vi "S2DS_Initial Scan parameters (SubVI).vi"(10 "Scan parameters (in)":T2 {"Y data taking" items=["in both direction", "in up direction only", "in down direction only"]; "X data taking" items=["in both direction", "in up direction only", "in down direction only"]}, 11 "WC info list":T3) -> (2 "WC Info list out":T1[](array[typedef]), 3 "Scan parameters out":T2 {"Y data taking" items=["in both direction", "in up direction only", "in down direction only"]; "X data taking" items=["in both direction", "in up direction only", "in down direction only"]})   [LabVIEW 2025]
uses:
  TYPE DEFS/S2DS_WC info.ctl
  TYPE DEFS/S2DS_Single WC info.ctl
  TYPE DEFS/S2DS_Sweep Info.ctl
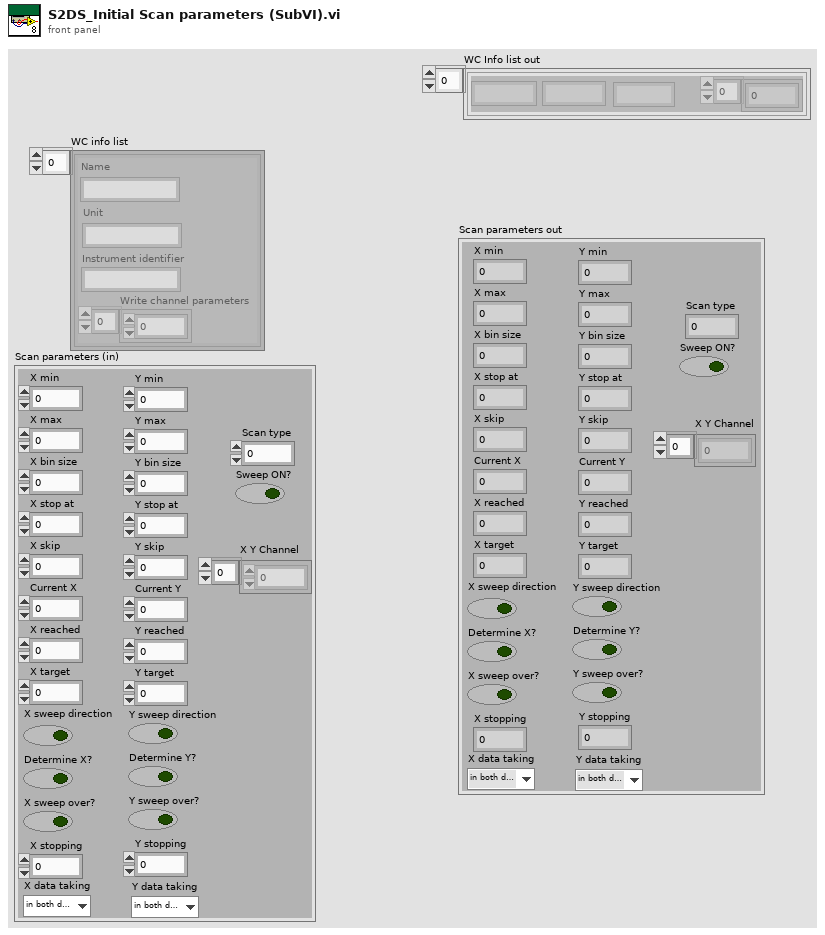
[diagram p1: front panel]
types:
  T1 = typedef "S2DS_Single WC info.ctl" = cluster{"Instrument identifier":string, "Write channel parameters":dbl[], "Name":string, "Unit":string}
  T2 = typedef "S2DS_Sweep Info.ctl" = cluster{"X min":ext, "X max":dbl, "Y min":dbl, "Y max":dbl, "X bin size":dbl, "Y bin size":dbl, "X stop at":dbl, "Y stop at":dbl, "X skip":u64, "Y skip":u64, "Current X":dbl, "Current Y":dbl, "X reached":i32, "Y reached":i32, "X target":dbl, "Y target":dbl, "Sweep ON?":bool, "X sweep direction":bool, "Y sweep direction":bool, "Determine X?":bool, "Determine Y?":bool, "X sweep over?":bool, "Y sweep over?":bool, "Scan type":i32, "X stopping":i32, "Y stopping":i32, "X Y Channel":u16[], "X data taking":u16, "Y data taking":u16}
  T3 = typedef "S2DS_WC info.ctl" = T1[]
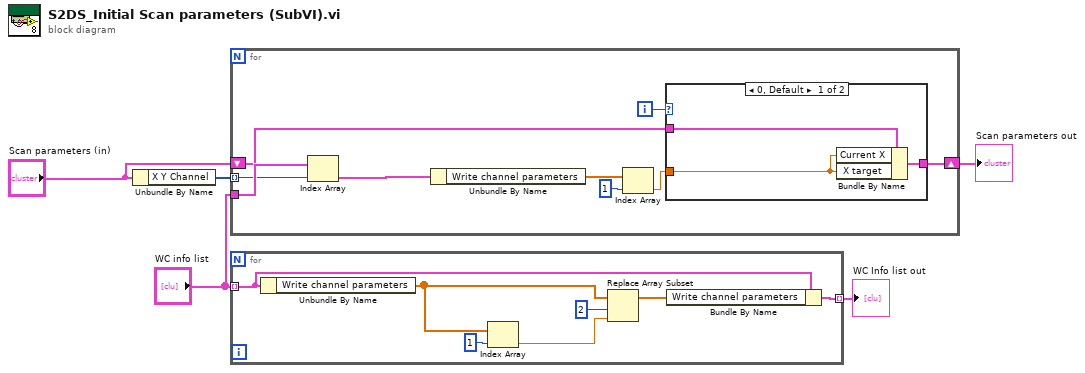
[diagram p0: block diagram]
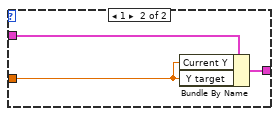
[diagram p2: hidden frame]
diagram:
  n1 = Unbundle By Name("Scan parameters (in)") -> ("X Y Channel"=w5:u16[])
  n2 = for {
    tunnel: w5 -> [w13] mode=indexing
    tunnel: "WC info list" -> [w14]
    shift-right: [w10] -> w3
    shift-left: "Scan parameters (in)" -> [w11]
    i -> [w12]
    n3 = Index Array(array=w14, index=w13) -> (element=w9:T1)
    n4 = Unbundle By Name(w9) -> ("Write channel parameters"=w8:dbl[])
    n5 = Index Array(array=w8, index=1) -> (element=w6:dbl)
    n6 = case shown="0, Default" w12 {
      tunnel: w11 -> [w17 w20]
      tunnel: [w16 w19] -> w10
      tunnel: w6 -> [w15 w18]
      frame 0, Default {
        n7 = Bundle By Name(cluster=w17, "Current X"=w15, "X target"=w15) -> (w16:T2)
      }
      frame 1 {
        n8 = Bundle By Name(cluster=w20, "Current Y"=w18, "Y target"=w18) -> (w19:T2)
      }
    }
  }
  "Scan parameters out" <- w3
  n9 = for {
    tunnel: "WC info list" -> [w27] mode=indexing
    tunnel: [w26] -> w1 mode=indexing
    n10 = Unbundle By Name(w27) -> ("Write channel parameters"=w24:dbl[])
    n11 = Index Array(array=w24, index=1) -> (element=w22:dbl)
    n12 = Replace Array Subset(array=w24, new element=w22, index=2) -> (w21:dbl[])
    n13 = Bundle By Name(cluster=w27, "Write channel parameters"=w21) -> (w26:T1)
  }
  "WC Info list out" <- w1
